vi "Close MeasurementLink Session.vi"(8 "error in":errorcluster, 9 "initialize and close session behavior":T1, 10 "session in":variant, 11 "session factory in":refnum<class "Session Factory.lvclass">) -> (0 "error out":errorcluster)   [LabVIEW 2021, in "NI Session Management niSE.lvlib" / "Session Factory.lvclass"]
doc: "Closes the local session. If the session represents a remote session, <b>initialize and close session behavior</b> determines whether closing the local session closes the server session or detaches from the server session."
uses:
  Session Factory.lvclass
  <vilib>/Plug-In SDKs/Sessions/Instrument/ISession Factory/Initialize and Close Session Behavior.ctl
  basic_switch_executive_driver_client/RPC Messages/nise_SessionInformation.ctl
  <vilib>/Plug-In SDKs/Clients/Session Management V1/Session Reservation/Initialize and Close Session Behavior.ctl
  Session Factory.lvclass/Session Factory.ctl
  basic_switch_executive_driver_client/basic_switch_executive_driver_client.lvlib
  <vilib>/Plug-In SDKs/Clients/Session Management V1/Session Reservation/Session Reservation.lvclass
  niSE simple relay - Disconnect/SimpleSwitch/SimpleSwitchDisconnect.lvlib
  <vilib>/Plug-In SDKs/Sessions/Instrument/ISession Factory/ISession Factory.lvclass
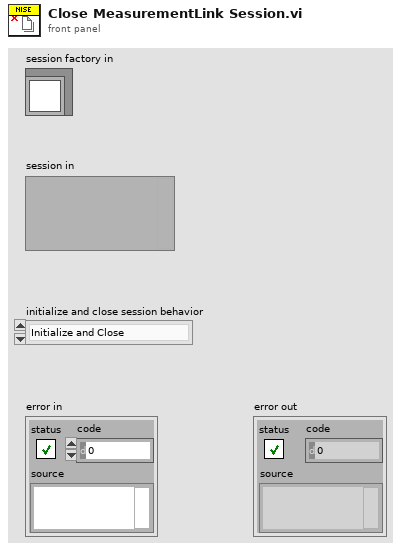
[diagram p1: front panel]
types:
  T1 = typedef "NI Session Management Instrument.lvlib/ISession Factory.lvclass/Initialize and Close Session Behavior.ctl" = enum16{"Initialize and Close", "Attach and Detach", "Initialize and Detach", "Attach and Close"}
  T2 = typedef "basic_switch_executive_driver_client.lvlib/nise_SessionInformation.ctl" = cluster{"session_id":u32, "initialize_and_close_session_behavior":T3}
  T3 = typedef "NI Session Management V1 Client.lvlib/Session Reservation.lvclass/Initialize and Close Session Behavior.ctl" = enum16{"Auto", "Initialize and Close", "Attach and Detach", "Initialize and Detach", "Attach and Close"}
  T4 = typedef "grpc-lvsupport-release.lvlib/grpcId.ctl" = u64
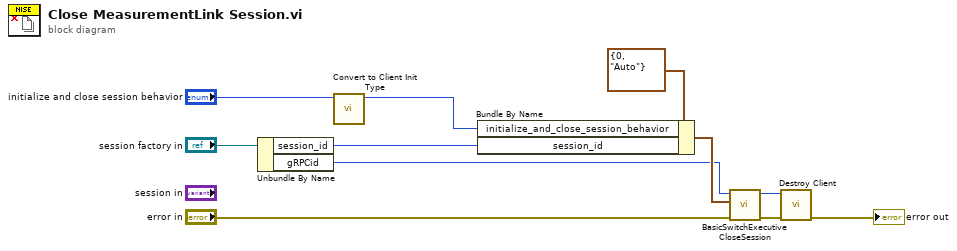
[diagram p0: block diagram]
diagram:
  n1 = Unbundle By Name("session factory in") -> ("session_id"=w4:u32, "gRPCid"=w1:T4)
  n2 = call "Convert to Client Init Type.vi"("initialize and close session behavior"="initialize and close session behavior") -> ("initialize_and_close_session_behavior"=w2:T3)  [unwired: 10 in]
  n3 = Bundle By Name(cluster=T2 {"session_id"=0, "initialize_and_close_session_behavior"=enum."Auto"} ("Request Data"), "initialize_and_close_session_behavior"=w2, "session_id"=w4) -> (w6:T2)
  n4 = call "BasicSwitchExecutive CloseSession.vi"("error in"="error in", "Request Data"=w6, "gRPC ID"=w1) -> ("error out"=w8:errorcluster, "gRPC ID out"=w7:T4)  [unwired: 6 in, 1 out]
  n5 = call "Destroy Client.vi"("error in"=w8, "gRPC ID"=w7) -> ("error out"=→"error out":errorcluster)  [unwired: 9 in]
